vi "RSNRPZ Two Sensor Connection.vi"(0 "Reset Device (T: Reset Device)":bool=TRUE, 1 "Resource Name 1 (USB::0xaad::0x00b::100000)":string="USB::0xaad::0x00b::100000", 5 "ID Query (T: Do Query)":bool=TRUE, 7 "Resource Name 2 (\"\")":string, 9 "Reset Device (T: Reset Device)":bool=TRUE, 11 "ID Query (T: Do Query)":bool=TRUE) -> (6 "Measurement Channel 1":dbl format="%.3p", 10 "Measurement Channel 2":dbl format="%.3p")   [LabVIEW 2010]
doc: "This VI runs two sensors measurement.\n- Open session to sensor specified by Resource Name\n- Initialize acqusistion, wait specified time for measurement and reads it."
panel:
  # "NRP-Z Power Meter\nTwo Sensor Measurement"
  # "Sensor 1"
  # "Sensor 2"
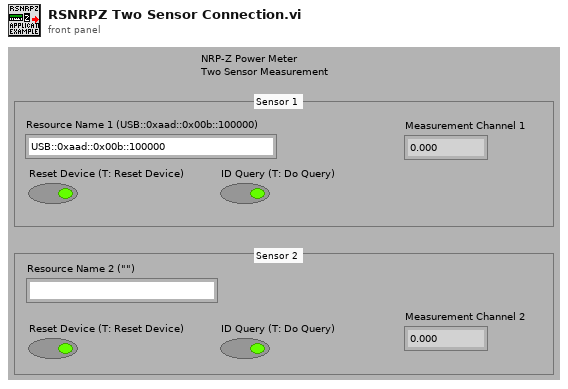
[diagram p1: front panel]
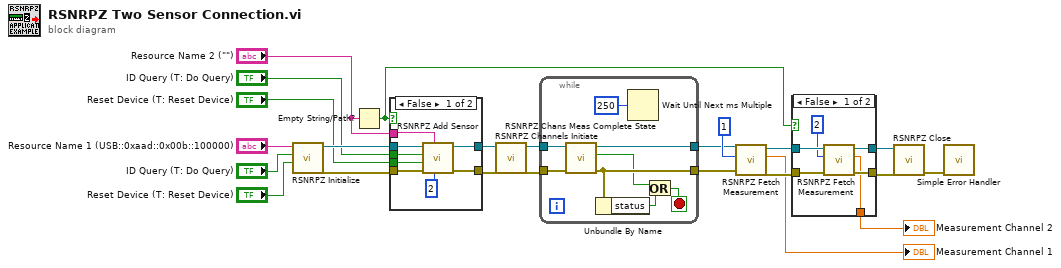
[diagram p0: block diagram]
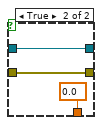
[diagram p2: hidden frame]
diagram:
  n1 = call <instrlib>:"RSNRPZ Initialize.vi"("Reset Device (T: Reset Device)"="Reset Device (T: Reset Device)", "ID Query (T: Do Query)"="ID Query (T: Do Query)", "Resource Name (USB::0x0aad::0x000b::100000)"="Resource Name 1 (USB::0xaad::0x00b::100000)") -> ("error out"=w18:errorcluster, "dup VISA session"=w19:refnum<visa-resource-name>)  [unwired: 7 in]
  n2 = Empty String/Path?(string/path="Resource Name 2 (\"\")") -> (empty?=w6:bool)
  n3 = case shown="False" w6 {
    tunnel: [w31 w33] -> w21
    tunnel: [w30 w32] -> w20
    tunnel: w19 -> [w29 w33]
    tunnel: w18 -> [w28 w32]
    tunnel: "Reset Device (T: Reset Device)" -> [w27 _]
    tunnel: "ID Query (T: Do Query)" -> [w25 _]
    tunnel: "Resource Name 2 (\"\")" -> [w24 _]
    frame False {
      n4 = call <instrlib>:"RSNRPZ Add Sensor.vi"("Channel (2)"=2, "Resource Name (USB::0xaad::0x00b::100000)"=w24, "error in (no error)"=w28, "Reset Device (T: Reset Device)"=w27, "ID Query (T: Do Query)"=w25, "VISA session"=w29) -> ("error out"=w30:errorcluster, "dup VISA session"=w31:refnum<visa-resource-name>)  [unwired: 4 in]
    }
    frame True {
    }
  }
  n5 = call <instrlib>:"RSNRPZ Channels Initiate.vi"("error in (no error)"=w20, "VISA session"=w21) -> ("error out"=w22:errorcluster, "dup VISA session"=w23:refnum<visa-resource-name>)  [unwired: 8 in]
  n6 = while {
    tunnel: w22 -> [w38]
    tunnel: w23 -> [w39]
    tunnel: [w40] -> w4
    tunnel: [w41] -> w3
    stop <- w35 stop-if-true
    n7 = call <instrlib>:"RSNRPZ Chans Meas Complete State.vi"("error in (no error)"=w38, "VISA session"=w39) -> ("error out"=w40:errorcluster, "Measurement Completed"=w36:bool, "dup VISA session"=w41:refnum<visa-resource-name>)  [unwired: 7 in]
    n8 = Unbundle By Name(w40) -> ("status"=w34:bool)
    n9 = Wait Until Next ms Multiple(millisecond multiple=u32 250) -> ()  [unwired: 1 out]
    n10 = Or(x=w36, y=w34) -> (x .or. y?=w35:bool)
  }
  n11 = call <instrlib>:"RSNRPZ Fetch Measurement.vi"("error in (no error)"=w4, "Channel (1)"=1, "VISA session"=w3) -> ("error out"=w17:errorcluster, "Measurement"=→"Measurement Channel 1":dbl, "dup VISA session"=w16:refnum<visa-resource-name>)  [unwired: 6 in]
  n12 = case shown="False" w6 {
    tunnel: w17 -> [w47 w50]
    tunnel: w16 -> [w46 w49]
    tunnel: [w44 w50] -> w2
    tunnel: [w43 w49] -> w15
    tunnel: [w42 0.0 ("Measurement")] -> w11
    frame False {
      n13 = call <instrlib>:"RSNRPZ Fetch Measurement.vi"("error in (no error)"=w47, "Channel (1)"=2, "VISA session"=w46) -> ("error out"=w44:errorcluster, "Measurement"=w42:dbl, "dup VISA session"=w43:refnum<visa-resource-name>)  [unwired: 6 in]
    }
    frame True {
    }
  }
  "Measurement Channel 2" <- w11
  n14 = call <instrlib>:"RSNRPZ Close.vi"("error in (no error)"=w2, "VISA session"=w15) -> ("error out"=w1:errorcluster)  [unwired: 9 in]
  n15 = call <vilib>:"Simple Error Handler.vi"("error in (no error)"=w1) -> ()  [unwired: 4 in, 5 out]
